vi "Clear.vi"(8 "error in (no error)":errorcluster, 11 "Gantry In":refnum<k24>) -> (0 "error out":errorcluster, 3 "Gantry Out":refnum<k24>)   [LabVIEW 2018, in "Motion.lvclass"]
uses:
  Motion.lvclass
  C:/Program Files (x86)/Aerotech/A3200/LabVIEW/2010/Bin/Aerotech.A3200.dll
  Program Files (x86)/Aerotech/A3200/LabVIEW/2010/Bin/Aerotech.A3200.dll
  A3200/A3200.lvclass
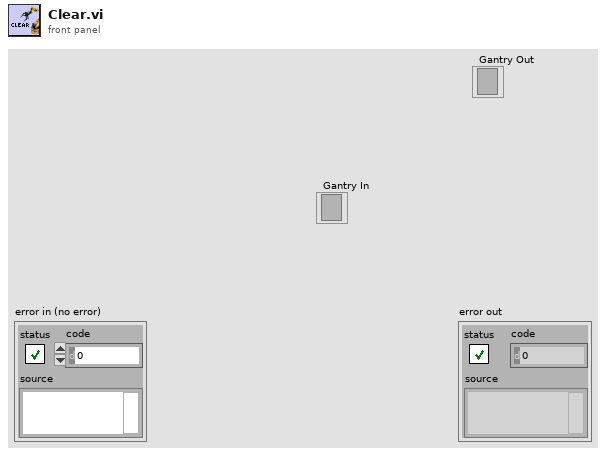
[diagram p1: front panel]
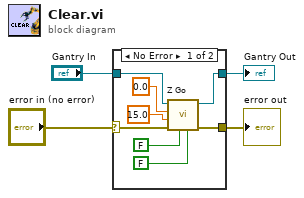
[diagram p0: block diagram]
diagram:
  n1 = case shown="No Error" "error in (no error)" {
    selector: "error in (no error)" -> [w7 w14]
    tunnel: [w6 w14] -> w3
    tunnel: [w9 w13] -> w1
    tunnel: "Gantry In" -> [w12 w13]
    frame No Error {
      n2 = call "Z Go.vi"("Increment"=FALSE, "Return Immediately"=FALSE ("Increment"), "error in (no error)"=w7, "Speed In"=15.0 ("Speed"), "Position In"=0.0 ("Position"), "Gantry In"=w12) -> ("error out"=w6:errorcluster, "Gantry Out"=w9:refnum<k24>)  [unwired: 2 in, 2 out]
    }
    frame Error {
    }
  }
  "error out" <- w3
  "Gantry Out" <- w1
